vi "Read I32.vi"(8 "error in (no error)":errorcluster, 11 "connection ID":refnum<k5>) -> (0 "error out":errorcluster, 2 "value":i32, 3 "connection ID out":refnum<k5>)   [LabVIEW 2014, in "Matlab API.lvlib"]
uses:
  Matlab API.lvlib
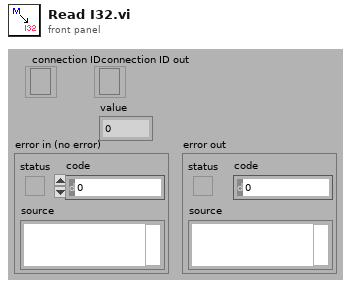
[diagram p1: front panel]
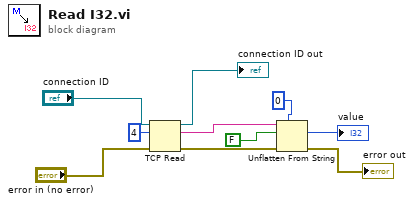
[diagram p0: block diagram]
diagram:
  n1 = TCP Read(connection ID="connection ID", bytes to read=4, error in (no error)="error in (no error)") -> (connection ID out=→"connection ID out":refnum<k5>, data out=w8:string, error out=w5:errorcluster)  [unwired: 2 out]
  n2 = Unflatten From String(type=0, binary string=w8, data includes array or string size? (T)=FALSE, error in (no error)=w5) -> (value=→"value":i32, error out=→"error out":errorcluster)  [unwired: 2 out]
